vi "CTRE_Phoenix_PigeonIMU_GetParameter.vi"(4 "ordinal":i32, 6 "timeoutMs":i32, 8 "error in":errorcluster, 10 "Parameter":T3=331 items=["eOnBoot_BrakeMode"=31, "eQuadFilterEn"=91, "eClearPositionOnIdx"=100, "eQuadIdxPolarity"=108, "eMotionProfileHasUnderrunErr"=119, "eMotionProfileTrajectoryPointDurationMs"=120, "eMotionProfileTrajectoryInterpolDis"=121, "eClearPosOnLimitF"=144, "eClearPosOnLimitR"=145, "eYawOffset"=160, "eCompassOffset"=161, "eBetaGain"=162, "eEnableCompassFustion"=163, "eGyroNoMotionCal"=164, "eEnterCalibration"=165, "eFusedHeadingOffset"=166, "eStatusFrameRate"=169, "eAccumZ"=170, "eTempCompDisable"=171, "eMotionMeas_tap_threshX"=172, "eMotionMeas_tap_threshY"=173, "eMotionMeas_tap_threshZ"=174, "eMotionMeas_tap_count"=175, "eMotionMeas_tap_time"=176, "eMotionMeas_tap_time_multi"=177, "eMotionMeas_shake_reject_thresh"=178, "eMotionMeas_shake_reject_time"=179, "eMotionMeas_shake_reject_timeout"=180, "eStatusFramePeriod"=300, "eOpenLoopRamp"=301, "eClosedLoopRamp"=302, "eNeutralDeadband"=303, "ePeakPosOutput"=305, "eNominalPosOutput"=306, "ePeakNegOutput"=307, "eNominalNegOutput"=308, "eProfileParamSlot_P"=310, "eProfileParamSlot_I"=311, "eProfileParamSlot_D"=312, "eProfileParamSlot_F"=313, "eProfileParamSlot_IZone"=314, "eProfileParamSlot_AllowableErr"=315, "eProfileParamSlot_MaxIAccum"=316, "eProfileParamSlot_PeakOutput"=317, "eClearPositionOnLimitF"=320, "eClearPositionOnLimitR"=321, "eClearPositionOnQuadIdx"=322, "eSampleVelocityPeriod"=325, "eSampleVelocityWindow"=326, "eFeedbackSensorType"=330, "eSelectedSensorPosition"=331, "eFeedbackNotContinuous"=332, "eRemoteSensorSource"=333, "eRemoteSensorDeviceID"=334, "eSensorTerm"=335, "eRemoteSensorClosedLoopDisableNeutralOnLOS"=336, "ePIDLoopPolarity"=337, "ePIDLoopPeriod"=338, "eSelectedSensorCoefficient"=339, "eForwardSoftLimitThreshold"=340, "eReverseSoftLimitThreshold"=341, "eForwardSoftLimitEnable"=342, "eReverseSoftLimitEnable"=343, "eNominalBatteryVoltage"=350, "eBatterVoltageFilterSize"=351, "eContinuousCurrentLimitAmps"=360, "eContinuousCurrentLimitMs"=361, "ePeakCurrentLimitAmps"=362, "eCurrEnable"=363, "eCurrThres_Ms"=364, "eClosedLoopIAccum"=370, "eCustomParam"=380, "eStickyFaults"=390, "eAnalogPosition"=400, "eQuadraturePosition"=401, "ePulseWidthPosition"=402, "eIntegratedSensor"=403, "eMotMag_Accel"=410, "eMotMag_VelCruise"=411, "eMotMag_SCurveLevel"=412, "eLimitSwitchSource"=421, "eLimitSwitchNormClosedAndDis"=422, "eLimitSwitchDisabledNeutralOnLOS"=423, "eLimitSwitchRemoteDevID"=424, "eSoftLimitDisabledNeutralOnLOS"=425, "ePulseWidthPeriod_EdgesPerRot"=430, "ePulseWidthPeriod_FilterWindowSz"=431, "eUnitString"=442, "eFeedbackTimeBase"=443, "eDefaultConfig"=500, "eFastWriteCount"=501, "eWriteCount"=502, "eReserved1"=555, "eMotorCommutation"=650, "eSensorInitStrategy"=700, "eSensorDirection"=701, "eMagnetOffset"=702, "eSensorSync"=703, "eAbsSensorRange"=704], 11 "PigeonIMUDevRef":T1={"DeviceStatus"={"status"=FALSE, "code"=0, "source"=""}, "Device Number"=0, "Type"=352321536, "Device ID"=0, "Handle"=0, "UsageFrame"=0, "Library Path"=path ""} {"Type" items=["CAN"=352321536, "TalonSRX"=33554432]}) -> (0 "error out":errorcluster, 2 "value":dbl, 3 "PigeonIMUDevRef":T1={"DeviceStatus"={"status"=FALSE, "code"=0, "source"=""}, "Device Number"=0, "Type"=352321536, "Device ID"=0, "Handle"=0, "UsageFrame"=0, "Library Path"=path ""} {"Type" items=["CAN"=352321536, "TalonSRX"=33554432]})   [LabVIEW 2020]
doc: "Returns the selected parameter value."
uses:
  <vilib>/Rock Robotics/WPI/ThirdParty/Phoenix-LabVIEW/Controls/CTRE_Phoenix_Params.ctl
  <vilib>/Rock Robotics/WPI/ThirdParty/Phoenix-LabVIEW/Pigeon IMU/CTRE_PigeonIMU_DeviceRef.ctl
  <vilib>/Rock Robotics/WPI/ThirdParty/Phoenix-LabVIEW/Pigeon IMU/CTRE_PigeonIMU_ConnectionType.ctl
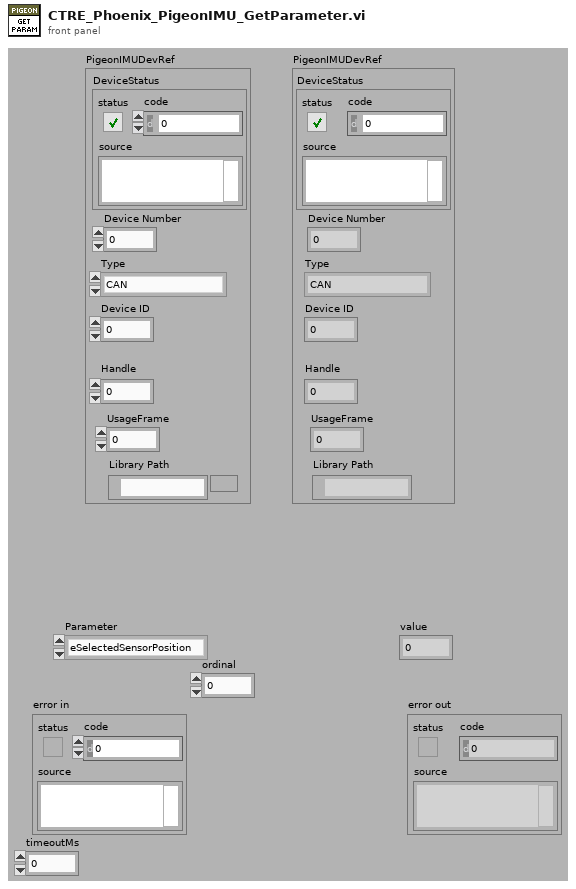
[diagram p1: front panel]
types:
  T1 = typedef "CTRE_PigeonIMU_DeviceRef.ctl" = cluster{"DeviceStatus":errorcluster, "Device Number":u8, "Type":T2, "Device ID":u32, "Handle":u64, "UsageFrame":u32, "Library Path":path}
  T2 = typedef "CTRE_PigeonIMU_ConnectionType.ctl" = u32
  T3 = typedef "CTRE_Phoenix_Params.ctl" = u16
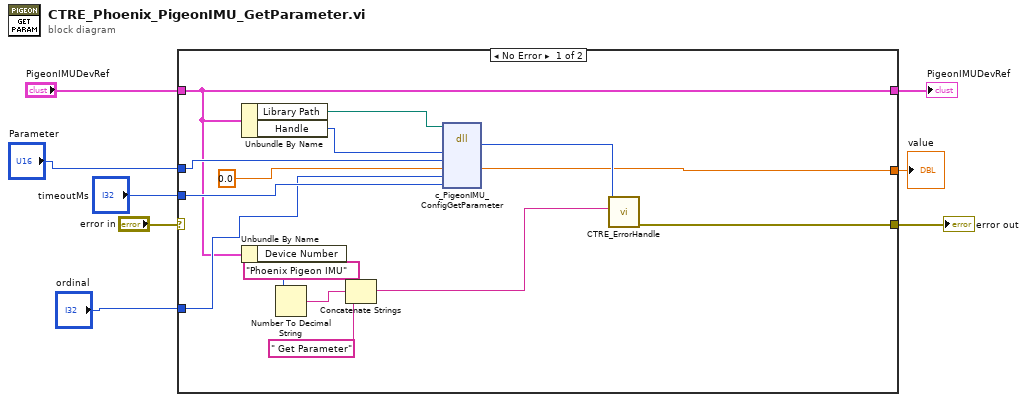
[diagram p0: block diagram]
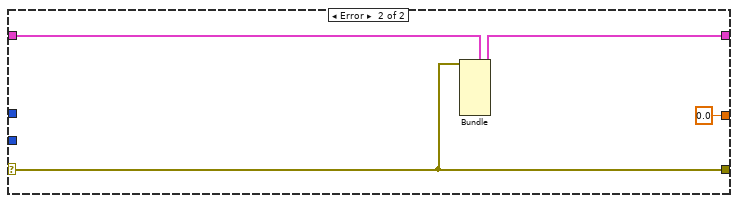
[diagram p2: hidden frame]
diagram:
  n1 = case shown="No Error" "error in" {
    selector: "error in" -> [_ w26]
    tunnel: "PigeonIMUDevRef" -> [w11 w27]
    tunnel: [w23 w26] -> w8
    tunnel: [w11 w25] -> w1
    tunnel: "Parameter" -> [w16 _]
    tunnel: [w14 sgl 0.0 ("value")] -> w5
    tunnel: "timeoutMs" -> [w13 _]
    tunnel: "ordinal" -> [w12 _]
    frame No Error {
      n2 = Unbundle By Name(w11) -> ("Library Path"=w10:path, "Handle"=w9:u64)
      n3 = Unbundle By Name(w11) -> ("Device Number"=w19:u8)
      n4 = Number To Decimal String(number=w19) -> (decimal integer string=w21:string)  [unwired: 1 in]
      n5 = Concatenate Strings("Phoenix Pigeon IMU" ("string"), w21, " Get Parameter" ("string")) -> (w17:string)
      n6 = dll-call lib="?" fn="c_PigeonIMU_ConfigGetParameter"(path in=w10, "handle"=w9, "param"=w16, "value"=0.0, "ordinal"=w12, "timeoutMs"=w13) -> ("return type"=w18:i32, "value"=w14:dbl)  [unwired: 6 in, 2 out]
      n7 = call <vilib>:"CTRE_ErrorHandle.vi"("origin"=w17, "code"=w18) -> ("error out"=w23:errorcluster)  [unwired: 9 in]
    }
    frame Error {
      n8 = Bundle(cluster=w27, "DeviceStatus"=w26) -> (w25:T1)  [unwired: 6 in]
    }
  }
  "error out" <- w8
  "value" <- w5
  "PigeonIMUDevRef" <- w1
